vi "Check Valid UI Selection.vi"(8 "error in (no error)":errorcluster, 11 "Operator UI in":refnum<class "Measurement UI.lvclass">) -> (0 "error out":errorcluster, 3 "Operator UI out":refnum<class "Measurement UI.lvclass">)   [LabVIEW 2017, in "Measurement UI.lvlib" / "Measurement UI.lvclass"]
uses:
  Measurement UI.lvclass
  Measurement UI.lvclass/Measurement UI.ctl
  Accessors/Read settings button array for hardware.vi
  Accessors/Read Run.vi
  Read Multimeter.vi
  Accessors/Read Digitizer.vi
  Accessors/Read Function Generator.vi
  Accessors/Read Show FP_.vi
  Accessors/Read Measurement.vi
  Read Step Config.vi
panel:
  out "Array":string[](array[string])
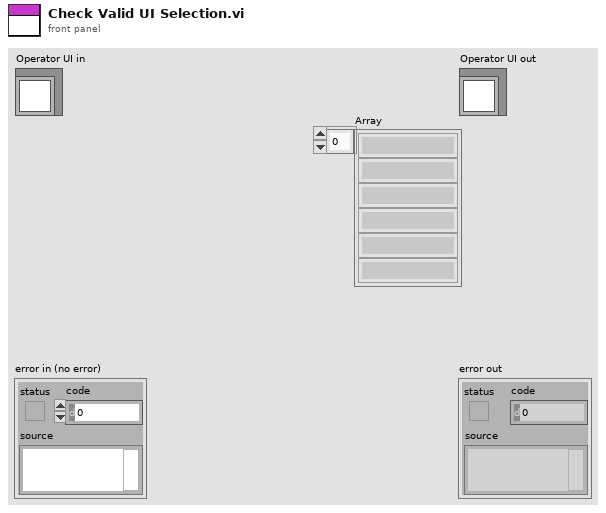
[diagram p1: front panel]
types:
  T1 = enum8{"Enabled", "Disabled", "Disabled and Grayed Out"}
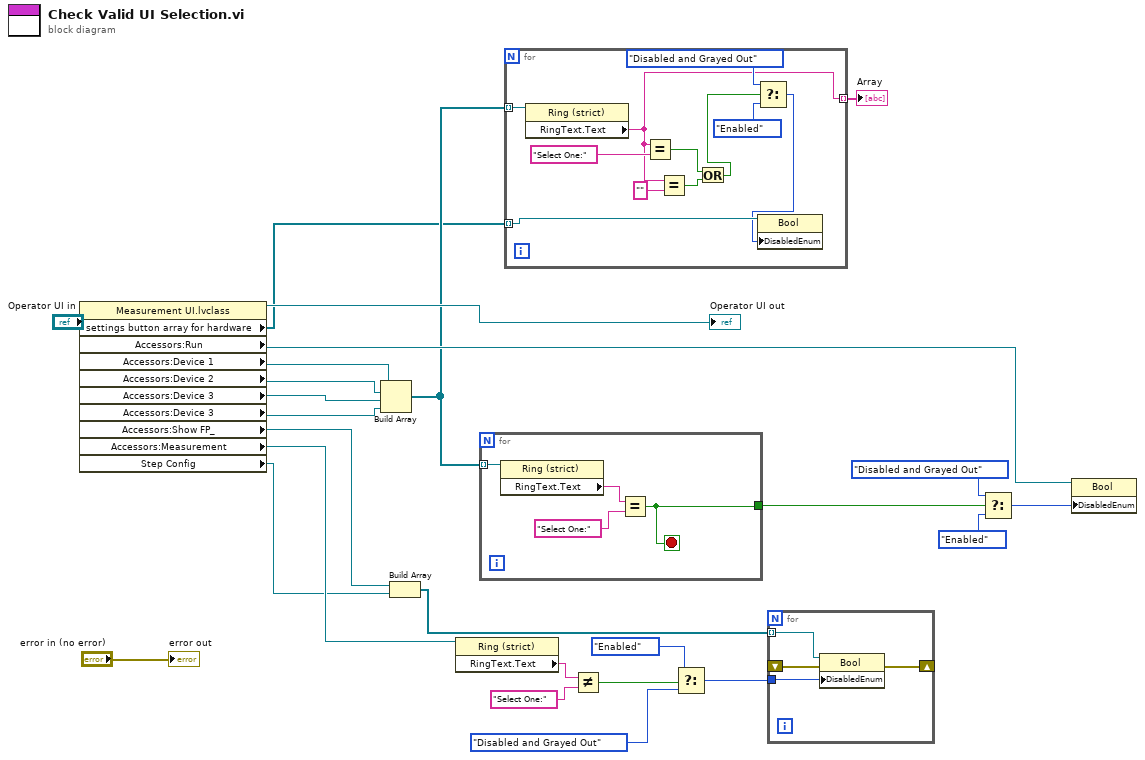
[diagram p0: block diagram]
diagram:
  n1 = property class="Measurement UI.lvclass"(reference="Operator UI in") -> (reference out=→"Operator UI out":refnum<class "Measurement UI.lvclass">, "settings button array for hardware"=w3:refnum<vi>[], "Accessors:Run"=w14:refnum<vi>, "Accessors:Device 1"=w15:refnum<vi>, "Accessors:Device 2"=w16:refnum<vi>, "Accessors:Device 3"=w17:refnum<vi>, "Accessors:Device 3"=w18:refnum<vi>, "Accessors:Show FP_"=w6:refnum<vi>, "Accessors:Measurement"=w7:refnum<vi>, "Step Config"=w1:refnum<vi>)  [unwired: 1 in, 1 out]
  n2 = Build Array(w15, w16, w17, w18) -> (w4:refnum<vi>[])
  n3 = Build Array(w6, w1) -> (w5:refnum<vi>[])
  n4 = property class="Ring (strict)"(reference=w7) -> ("RingText.Text"=w13:string)  [unwired: 1 in, 2 out]
  n5 = for {
    tunnel: w4 -> [w29] mode=indexing
    tunnel: [w26] -> w22
    stop <- w26 stop-if-true
    n6 = property class="Ring (strict)"(reference=w29) -> ("RingText.Text"=w28:string)  [unwired: 1 in, 2 out]
    n7 = Equal?(x=w28, y="Select One:") -> (x = y?=w26:bool)
  }
  n8 = for {
    tunnel: w4 -> [w40] mode=indexing
    tunnel: w3 -> [w39] mode=indexing
    tunnel: [w34] -> w2 mode=indexing
    n9 = property class="Ring (strict)"(reference=w40) -> ("RingText.Text"=w34:string)  [unwired: 1 in, 2 out]
    n10 = Equal?(x=w34, y="Select One:") -> (x = y?=w31:bool)
    n11 = Equal?(x=w34, y="") -> (x = y?=w32:bool)
    n12 = Or(x=w31, y=w32) -> (x .or. y?=w30:bool)
    n13 = Select(t=T1."Disabled and Grayed Out" ("Disabled"), s=w30, f=T1."Enabled" ("Disabled")) -> (s? t:f=w36:T1)
    n14 = property class="Bool"(reference=w39, "DisabledEnum"=w36) -> ()  [unwired: 1 in, 2 out]
  }
  "Array" <- w2
  n15 = Not Equal?(x=w13, y="Select One:") -> (x != y?=w11:bool)
  n16 = Select(t=T1."Enabled" ("Disabled"), s=w11, f=T1."Disabled and Grayed Out" ("Disabled")) -> (s? t:f=w8:T1)
  n17 = for {
    tunnel: w8 -> [w44]
    tunnel: w5 -> [w43] mode=indexing
    shift-right: [w42] -> _
    shift-left: _ -> [w41]
    n18 = property class="Bool"(reference=w43, error in=w41, "DisabledEnum"=w44) -> (error out=w42:errorcluster)  [unwired: 1 out]
  }
  n19 = Select(t=T1."Disabled and Grayed Out" ("Disabled"), s=w22, f=T1."Enabled" ("Disabled")) -> (s? t:f=w23:T1)
  n20 = property class="Bool"(reference=w14, "DisabledEnum"=w23) -> ()  [unwired: 1 in, 2 out]
  "error out" <- "error in (no error)"
